vi "Check.vi"(7 "VolatusAPI":refnum<class "VolatusAPI.lvclass">, 8 "error in (no error)":errorcluster, 11 "EStop Source in":refnum<class "EStop Source.lvclass">) -> (0 "error out":errorcluster, 3 "EStop Source out":refnum<class "EStop Source.lvclass">)   [LabVIEW 2020, in "VolatusControl.lvlib" / "EStop Source.lvclass"]
uses:
  EStop Source.lvclass
  Volatus/VolatusAPI/VolatusAPI.lvclass
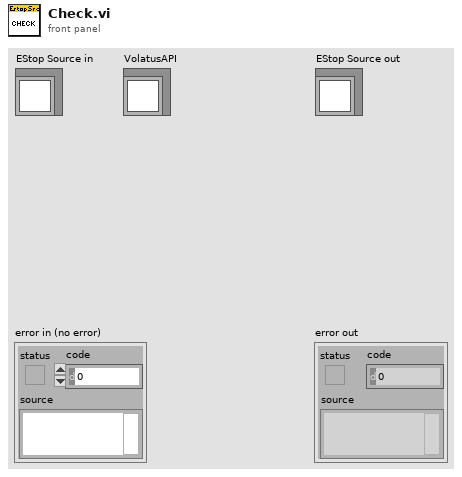
[diagram p1: front panel]
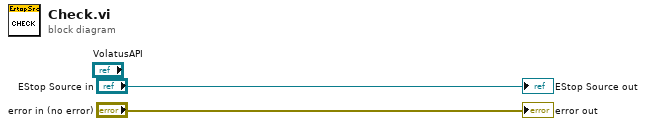
[diagram p0: block diagram]
diagram:
  "error out" <- "error in (no error)"
  "EStop Source out" <- "EStop Source in"
